vi "Read Multi Eval Meas SEM Results.vi"(8 "error in (no error)":errorcluster, 9 "Result Type (Current)":i32(ring) items=["Current"=0, "Average"=1, "Standard Deviation"=3], 10 "Instance (1)":T2=1, 11 "VISA resource name":refnum<visa-resource-name>) -> (0 "error out":errorcluster, 1 "SEM Results":T1 {"TX Power" format="%^.3e"; "Occupied Bandwidth" format="%^.3e"}, 2 "Reliability":i32, 3 "VISA resource name out":refnum<visa-resource-name>, 5 "Out Of Tolerance":i32)   [LabVIEW 2020, in "Rohde&Schwarz CMWXP NR FR1 Measurement.lvlib"]
doc: "Return the current, average and standard deviation single value results of the spectrum emission measurement.\n\nAttributes:\nRSCMWXPNRFR1M_ATTR_READ_MULTI_EVAL_MEAS_SEM_CURRENT_RESULTS\nRSCMWXPNRFR1M_ATTR_READ_MULTI_EVAL_MEAS_SEM_AVERAGE_RESULTS\nRSCMWXPNRFR1M_ATTR_READ_MULTI_EVAL_MEAS_SEM_STANDARD_DEVIATION_RESULTS\n\nRemote-control commands:\nREAD:NRSub:MEAS<i>:MEValuation:SEMask:CURRent?\nREAD:NRSub:MEAS<i>:MEValuation:SEMask:AVERage?\nREAD:NRSub:MEAS<i>:MEValuation:SEMask:SDEViation?"
uses:
  <instrlib>/Rohde&Schwarz CMWXP NR FR1 Measurement/Rohde&Schwarz CMWXP NR FR1 Measurement.lvlib
  <instrlib>/Rohde&Schwarz CMWXP NR FR1 Measurement/Private/_Instance.ctl
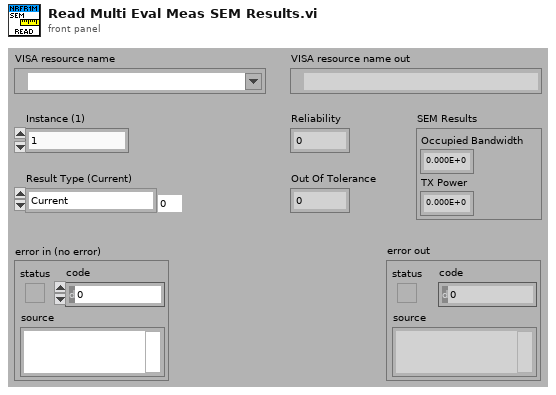
[diagram p1: front panel]
types:
  T1 = cluster{"Occupied Bandwidth":dbl, "TX Power":dbl}
  T2 = typedef "Rohde&Schwarz CMWXP NR FR1 Measurement.lvlib/_Instance.ctl" = i32
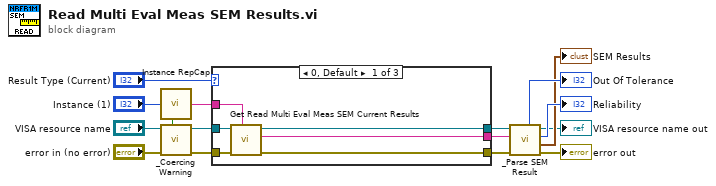
[diagram p0: block diagram]
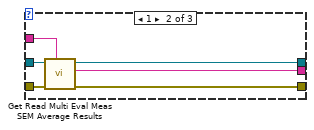
[diagram p2: hidden frame]
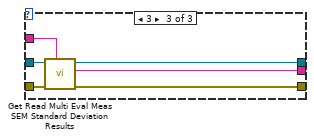
[diagram p3: hidden frame]
diagram:
  n1 = call <instrlib>:"Instance RepCap.vi"("Instance In"="Instance (1)") -> ("In Range?"=w13:bool, "RepCap Identifier Out"=w10:string)  [unwired: 1 in]
  n2 = call <instrlib>:"_Coercing Warning.vi"("In Range?"=w13, "error in (no error)"="error in (no error)", "VISA resource name"="VISA resource name") -> ("error out"=w11:errorcluster, "VISA resource name out"=w12:refnum<visa-resource-name>)  [unwired: 7 in]
  n3 = case shown="0, Default" "Result Type (Current)" {
    tunnel: w12 -> [w22 w28 w34]
    tunnel: w11 -> [w21 w27 w33]
    tunnel: w10 -> [w20 w26 w32]
    tunnel: [w19 w25 w31] -> w8
    tunnel: [w18 w24 w30] -> w7
    tunnel: [w17 w23 w29] -> w6
    frame 0, Default {
      n4 = call "Get Read Multi Eval Meas SEM Current Results"("Repeated Capabilities"=w20, "error in (no error)"=w21, "instrument handle"=w22) -> ("error out"=w17:errorcluster, "Read Multi Eval Meas SEM Current Results"=w18:string, "instrument handle out"=w19:refnum<visa-resource-name>)  [unwired: 6 in]
    }
    frame 1 {
      n5 = call "Get Read Multi Eval Meas SEM Average Results"("Repeated Capabilities"=w26, "error in (no error)"=w27, "instrument handle"=w28) -> ("error out"=w23:errorcluster, "Read Multi Eval Meas SEM Average Results"=w24:string, "instrument handle out"=w25:refnum<visa-resource-name>)  [unwired: 6 in]
    }
    frame 3 {
      n6 = call "Get Read Multi Eval Meas SEM Standard Deviation Results"("Repeated Capabilities"=w32, "error in (no error)"=w33, "instrument handle"=w34) -> ("error out"=w29:errorcluster, "Read Multi Eval Meas SEM Standard Deviation Results"=w30:string, "instrument handle out"=w31:refnum<visa-resource-name>)  [unwired: 6 in]
    }
  }
  n7 = call <instrlib>:"_Parse SEM Result.vi"("error in (no error)"=w6, "Input String"=w7, "VISA resource name"=w8) -> ("error out"=→"error out":errorcluster, "SEM Results"=→"SEM Results":T1, "Reliability"=→"Reliability":i32, "VISA resource name out"=→"VISA resource name out":refnum<visa-resource-name>, "Out Of Tolerance"=→"Out Of Tolerance":i32)  [unwired: 4 in]
